vi "Wristband main - Keytap Leap based.vi"() -> ()   [LabVIEW 2014]
uses:
  Typedef/sensor_data.ctl
  Typedef/keytap_data.ctl
  Typedef/flexext_data.ctl
  SubVIs/Save Blocks - 2D.vi
  <vilib>/MakerHub/LINX/Public/Peripherals/Analog/Analog Read N Chans.vi
  <vilib>/MakerHub/LINX/LMH-LINX.lvlib
panel:
  in  "X Scale.Range:Maximum":dbl=200.0 format="%#_13g"
  in  "X Scale.Range:Minimum":dbl format="%#_13g"
  in  "X-scale change":bool
  in  "Clear Plot":bool
  in  "Acquire":bool
  in  "Tacq":u32=50 caption="Acquisition Interval" min=50 max=10000 step=50 format="%.0fms"
  in  "N pts":i32=500
  in  "Session name":string="Sessione Mat"
  in  "Save to path":path=path "C:/Users/Andrea/Desktop/Programmi LabView/Smart Wristband"
  out "Leap \nConnected?":bool caption="Leap Motion"
  in  "Arduino Port":refnum<visa-resource-name>="COM4"
  out "Status":bool=TRUE caption="Arduino"
  out "Sensor Chart":T1(graph)
  out "Grab Strength":u8
  out "Flexext cluster":T2
  out "Keytap cluster":T3={"Pollice"=5, "Indice"=5, "Medio"=5, "Anulare"=5, "Mignolo"=5}
  out "Sensor Data":T4={"Sensor  Chan 0"=1.66015625, "Sensor Chan 1"=2.060546875, "Sensor Chan 2"=2.099609375, "Sensor Chan 3"=2.12890625, "Sensor Chan 4"=2.0751953125, "Sensor Chan 5"=1.8115234375}
  in  "Exit":bool=TRUE
  out "Event Chart":T5(graph)={"Estensione"=0, "Flessione"=0, "Pollice"=5, "Indice"=5, "Medio"=5, "Anulare"=5, "Mignolo"=5, "Grab Strength"=0}
  # "Connection panel"
  # "Acquisition panel"
  # "Save settings"
  # "Connection status"
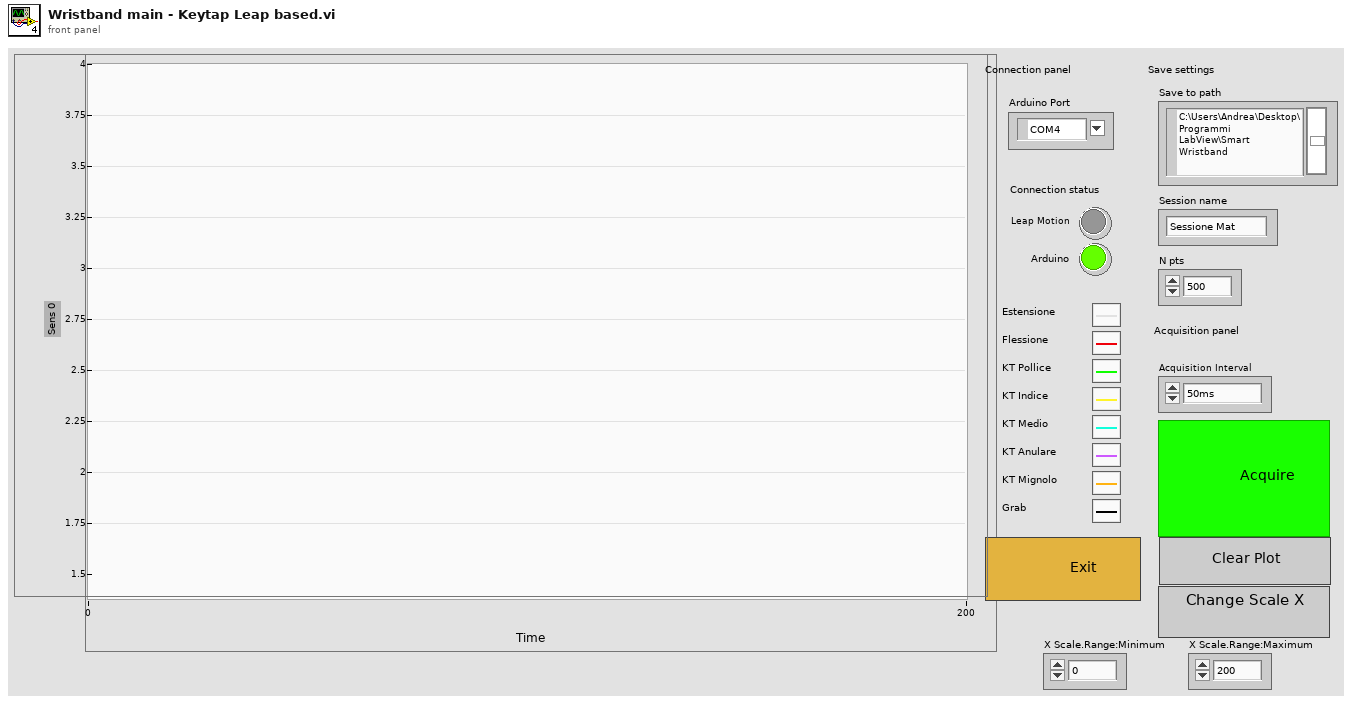
[diagram p1: front panel]
types:
  T1 = cluster{"Sensor  Chan 0":dbl, "Sensor Chan 2":dbl, "Sensor Chan 4":dbl, "Sensor Chan 5":dbl}
  T2 = typedef "flexext_data.ctl" = cluster{"Estensione":u8, "Flessione":u8}
  T3 = typedef "keytap_data.ctl" = cluster{"Pollice":u8, "Indice":u8, "Medio":u8, "Anulare":u8, "Mignolo":u8}
  T4 = typedef "Sensor_data.ctl" = cluster{"Sensor  Chan 0":dbl, "Sensor Chan 1":dbl, "Sensor Chan 2":dbl, "Sensor Chan 3":dbl, "Sensor Chan 4":dbl, "Sensor Chan 5":dbl}
  T5 = cluster{"Estensione":u8, "Flessione":u8, "Pollice":u8, "Indice":u8, "Medio":u8, "Anulare":u8, "Mignolo":u8, "Grab Strength":u8}
  T6 = typedef "LMH-LINX.lvlib/LINX Ref.ctl" = cluster{"Platform":T7, "Interface":T8, "LINX Device Config":T9}
  T7 = typedef "LMH-LINX.lvlib/Platform.ctl" = enum16{"LINX", "myRIO"}
  T8 = typedef "LMH-LINX.lvlib/Interface.ctl" = enum16{"Serial", "TCP"}
  T9 = typedef "LMH-LINX.lvlib/Device.lvlib/LINX Device Config.ctl" = cluster{"Interface":T8, "COM Port":refnum<visa-resource-name>, "TCP Configuration":T10, "Device Family":u8, "Device ID":u8, "Device Name":string, "TCP Ref":refnum<k5>, "Channels":T11}
  T10 = typedef "LMH-LINX.lvlib/Device.lvlib/TCP Config.ctl" = cluster{"IP Address":string, "Port":u16}
  T11 = typedef "LMH-LINX.lvlib/Channels.ctl" = cluster{"DI":u8[], "DO":u8[], "AI":u8[], "AO":u8[], "PWM":u8[], "QE":u8[], "UART":u8[], "I2C 2":u8[], "SPI":u8[], "CAN":u8[], "Servo":u8[], "AI Ref (V)":dbl, "AO Ref (V)":dbl, "AO Resolution (Bits)":u8}
  T12 = typedef "Leap Handle.ctl" = cluster{"LeapCSharp":refnum<k24>}
  T13 = cluster{"Estensione":u8, "Flessione":u8, "Pollice":u8, "Indice":u8, "Medio":u8, "Anulare":u8, "Mignolo":u8, "Grab Strength":u8}[]
  T14 = cluster{"Sensor  Chan 0":dbl, "Sensor Chan 2":dbl, "Sensor Chan 4":dbl, "Sensor Chan 5":dbl}[]
  T15 = cluster{"Sensor  Chan 0":dbl, "Sensor Chan 1":dbl, "Sensor Chan 2":dbl, "Sensor Chan 3":dbl}
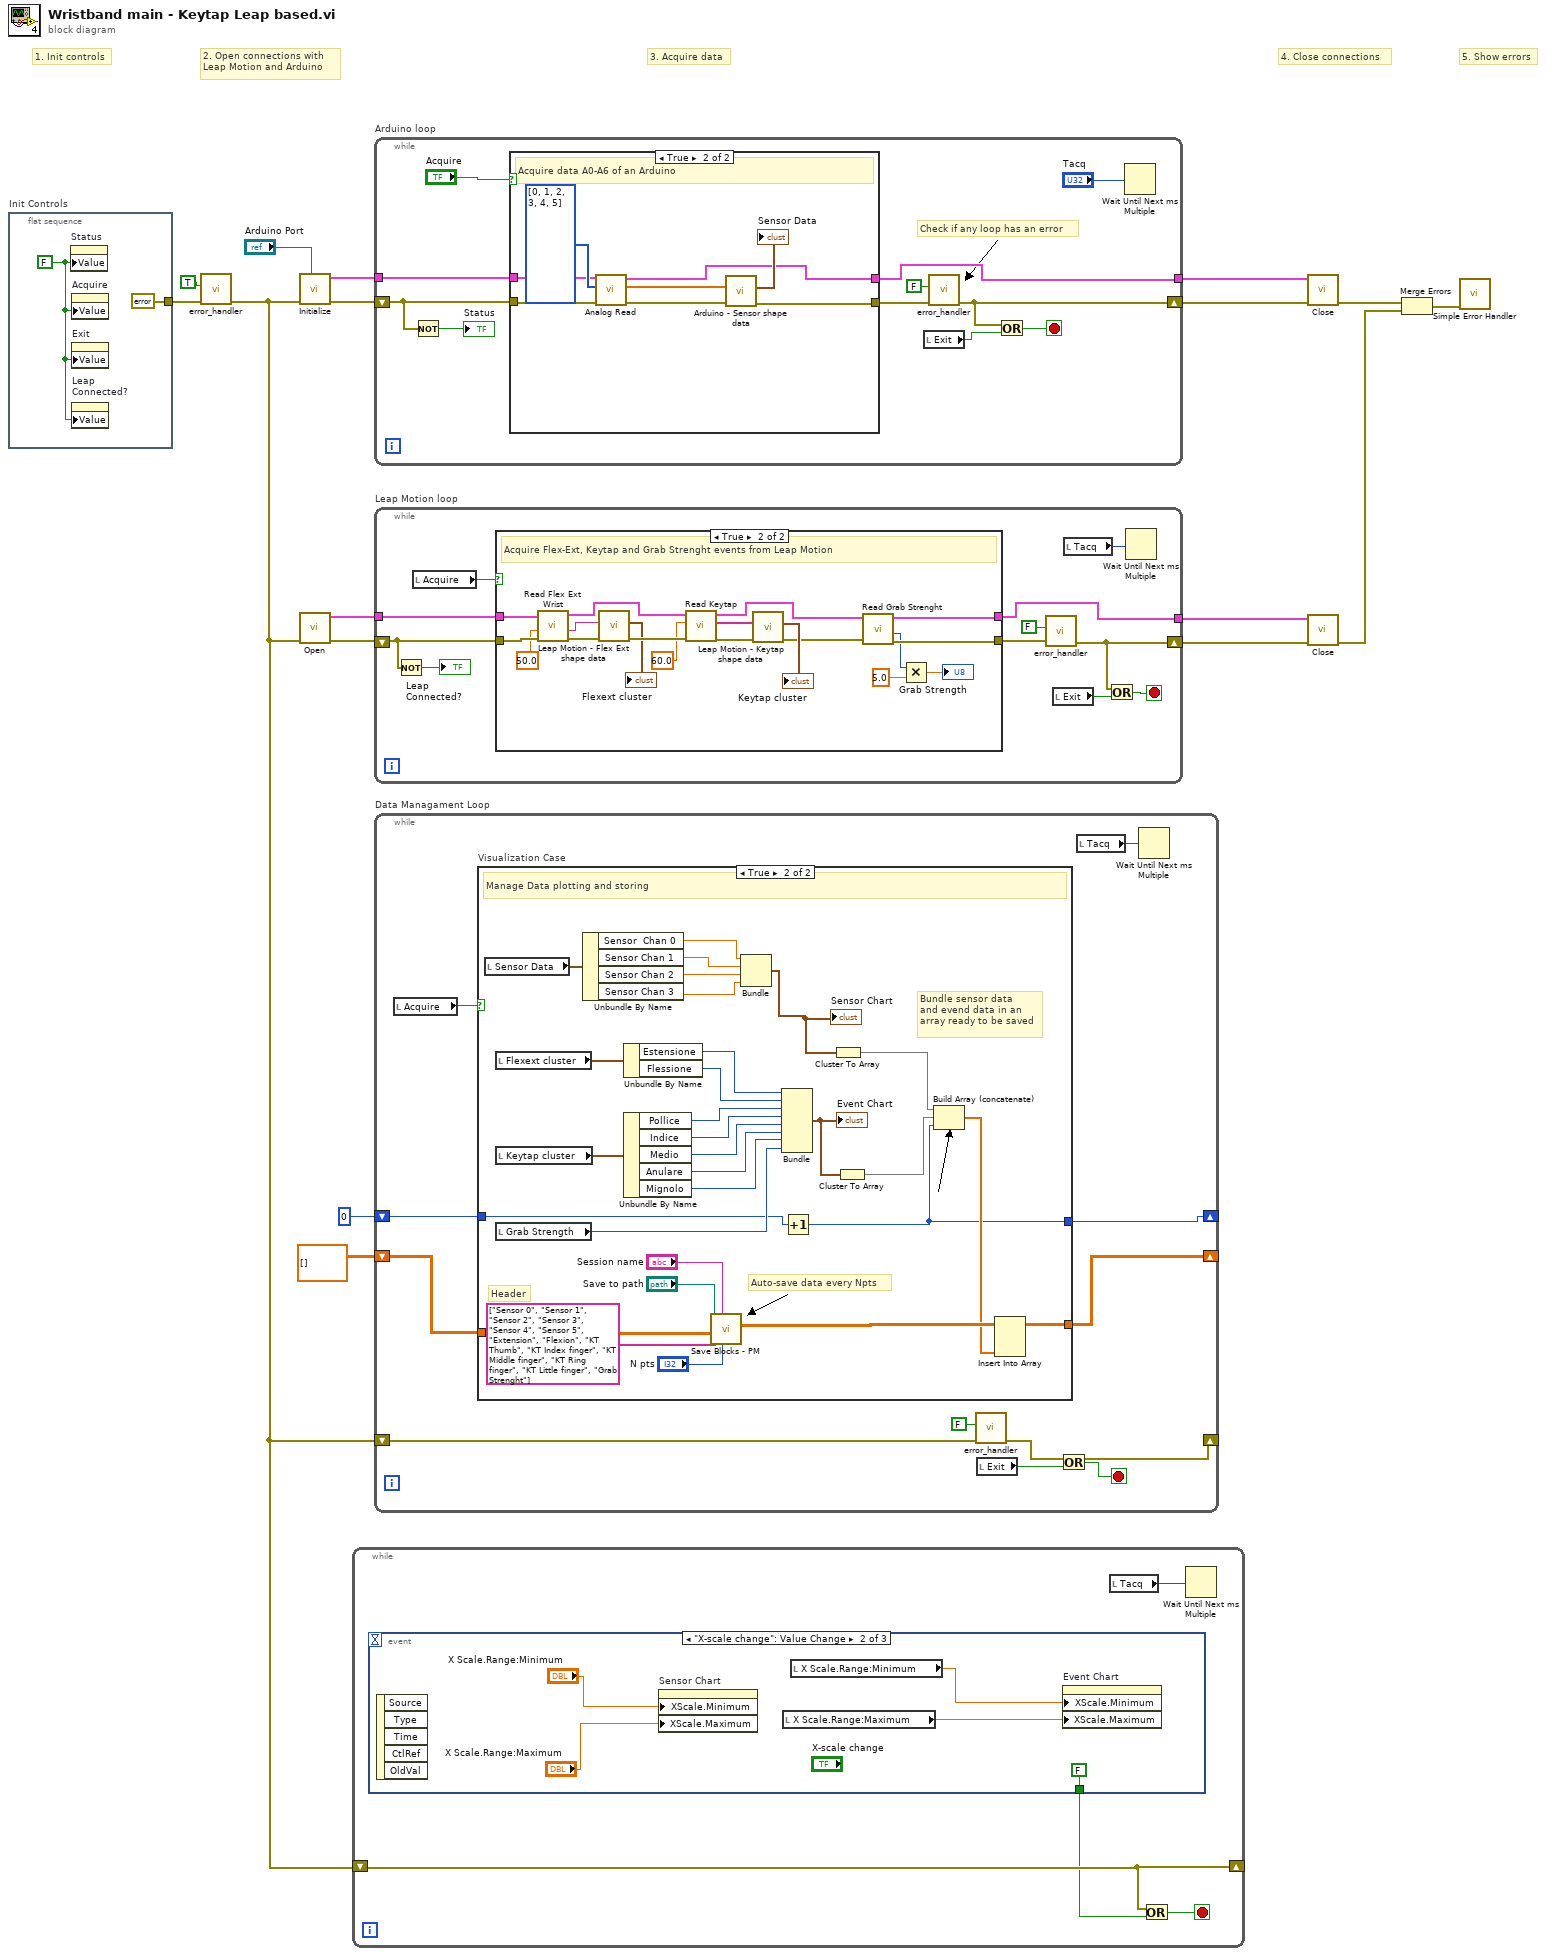
[diagram p0: block diagram]
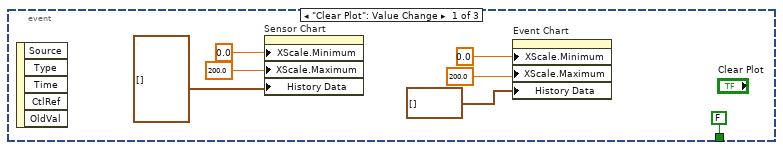
[diagram p2: hidden frame]
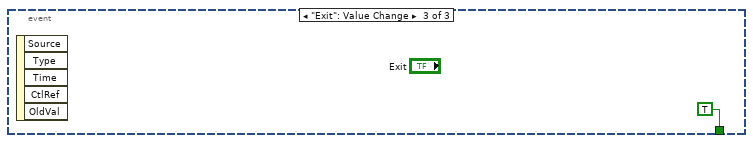
[diagram p3: hidden frame]
diagram:
  # "5. Show errors"
  # "4. Close connections"
  # "3. Acquire data"
  # "2. Open connections with\nLeap Motion and Arduino"
  # "1. Init controls"
  n1 = flat-sequence "Init Controls" {
    tunnel: [errorcluster {"status"=FALSE, "code"=0, "source"=""} ("Error In")] -> w8
    frame #0 {
      w18 = FALSE ("Status")
      n2 = property on="Status" class="Bool (strict)"("Value"=w18) -> ()  [unwired: 2 in, 2 out]
      n3 = property on="Acquire" class="Bool (strict)"("Value"=w18) -> ()  [unwired: 2 in, 2 out]
      n4 = property on="Exit" class="Bool (strict)"("Value"=w18) -> ()  [unwired: 2 in, 2 out]
      n5 = property on="Leap \nConnected?" class="Bool (strict)"("Value"=w18) -> ()  [unwired: 2 in, 2 out]
    }
  }
  n6 = call "error_handler.vi"("Error In"=w8, "Reset"=TRUE) -> ("Error Out"=w2:errorcluster)  [unwired: 9 in]
  n7 = call <vilib>:"Initialize.vi"("Serial Port"="Arduino Port", "Error In"=w2) -> ("Error Out"=w16:errorcluster, "LINX Ref"=w17:T6)  [unwired: 7 in, 1 out]
  n8 = call "Open.vi"("Error In"=w2) -> ("Error Out"=w11:errorcluster, "Leap Handle"=w12:T12)  [unwired: 9 in]
  n9 = while {
    shift-right: [w21] -> _
    shift-left: w2 -> [w21]
    stop <- w22 stop-if-true
    n10 = event shown="[1] \"X-scale change\": Value Change" {
      selector: _ -> [_ _ _]
      dyn-events: _ -> [_ _ _]
      timeout: _ -> [_ _ _]
      tunnel: [FALSE FALSE TRUE] -> w20
      event "Clear Plot": Value Change {
        n11 = event-data() -> ()  [unwired: 1 in, 5 out]
        n12 = property on="Sensor Chart" class="WFChart (strict)"("XScale.Minimum"=0.0 ("X Scale.Range:Minimum"), "XScale.Maximum"=200.0 ("X Scale.Range:Maximum"), "History Data"=T14 []) -> ()  [unwired: 2 in, 2 out]
        n13 = property on="Event Chart" class="WFChart (strict)"("XScale.Minimum"=0.0 ("X Scale.Range:Minimum"), "XScale.Maximum"=200.0 ("X Scale.Range:Maximum"), "History Data"=T13 []) -> ()  [unwired: 2 in, 2 out]
      }
      event "X-scale change": Value Change {
        n14 = event-data() -> ()  [unwired: 1 in, 5 out]
        n15 = property on="Sensor Chart" class="WFChart (strict)"("XScale.Minimum"="X Scale.Range:Minimum", "XScale.Maximum"="X Scale.Range:Maximum") -> ()  [unwired: 2 in, 2 out]
        n16 = local read "X Scale.Range:Maximum"() -> (w31:dbl)
        n17 = local read "X Scale.Range:Minimum"() -> (w34:dbl)
        n18 = property on="Event Chart" class="WFChart (strict)"("XScale.Minimum"=w34, "XScale.Maximum"=w31) -> ()  [unwired: 2 in, 2 out]
      }
      event "Exit": Value Change {
        n19 = event-data() -> ()  [unwired: 1 in, 5 out]
      }
    }
    n20 = local read "Tacq"() -> (w23:u32)
    n21 = Or(x=w21, y=w20) -> (x .or. y?=w22:bool)
    n22 = Wait Until Next ms Multiple(millisecond multiple=w23) -> ()  [unwired: 1 out]
  }
  n23 = while "Arduino loop" {
    tunnel: w17 -> [w46]
    tunnel: [w39] -> w13
    shift-right: [w40] -> w14
    shift-left: w16 -> [w43]
    stop <- w45 stop-if-true
    # "Check if any loop has an error"
    n24 = Not(x=w43) -> (.not. x?=→"Status":bool)
    n25 = case shown="True" "Acquire" {
      tunnel: w46 -> [w48 w55]
      tunnel: w43 -> [w49 w57]
      tunnel: [w48 w50] -> w39
      tunnel: [w49 w53] -> w41
      frame False {
        # "Idle"
      }
      frame True {
        # "Acquire data A0-A6 of an Arduino"
        n26 = call-poly <vilib>:"Analog Read.vi"("Error In"=w57, "AI Channel(s)"=u8[] [0, 1, 2, 3, 4, 5], "LINX Resource"=w55) -> ("Error Out"=w54:errorcluster, "Voltages"=w52:dbl[], "LINX Resource"=w50:T6)  [unwired: 5 in, 1 out]
        n27 = call "Arduino - Sensor shape data.vi"("Error In"=w54, "Sensor Data in"=w52) -> ("Error Out"=w53:errorcluster, "Sensor Data Out"=→"Sensor Data":T4)  [unwired: 8 in]
      }
    }
    n28 = local read "Exit"() -> (w37:bool)
    n29 = call "error_handler.vi"("Error In"=w41, "Reset"=FALSE) -> ("Error Out"=w40:errorcluster)  [unwired: 9 in]
    n30 = Or(x=w40, y=w37) -> (x .or. y?=w45:bool)
    n31 = Wait Until Next ms Multiple(millisecond multiple="Tacq") -> ()  [unwired: 1 out]
  }
  n32 = while "Leap Motion loop" {
    tunnel: w12 -> [w66]
    tunnel: [w60] -> w10
    shift-right: [w62] -> w9
    shift-left: w11 -> [w59]
    stop <- w67 stop-if-true
    n33 = Not(x=w59) -> (.not. x?=→"Leap \nConnected?":bool)
    n34 = local read "Acquire"() -> (w64:bool)
    n35 = case shown="True" w64 {
      tunnel: w66 -> [w70 w89]
      tunnel: w59 -> [w69 w88]
      tunnel: [w70 w76] -> w60
      tunnel: [w69 w75] -> w63
      frame False {
        # "Idle"
      }
      frame True {
        # "Acquire Flex-Ext, Keytap and Grab Strenght events from Leap Motion"
        n36 = call "Read Flex Ext Wrist.vi"("Error In"=w88, "Flex Extension threshold"=sgl 50.0, "Leap Handle In"=w89) -> ("Error Out"=w86:errorcluster, "Wrist Flextion/Extension"=w85:string, "Leap Handle Out"=w84:T12)  [unwired: 4 in]
        n37 = call "Leap Motion - Flex Ext shape data.vi"("Error In"=w86, "Event In"=w85) -> ("Error Out"=w83:errorcluster, "Flexext cluster"=→"Flexext cluster":T2)  [unwired: 8 in]
        n38 = call "Read Keytap.vi"("Error In"=w83, "Key Tap Thresh"=sgl 60.0, "Leap Handle In"=w84) -> ("Error Out"=w82:errorcluster, "Key tap"=w81:string[], "Leap Handle Out"=w78:T12)  [unwired: 3 in, 2 out]
        n39 = call "Leap Motion - Keytap shape data.vi"("Error In"=w82, "Key tap"=w81) -> ("Error Out"=w77:errorcluster, "Keytap cluster"=→"Keytap cluster":T3)  [unwired: 8 in]
        n40 = call "Read Grab Strenght.vi"("Error In"=w77, "Leap Handle In"=w78) -> ("Error Out"=w75:errorcluster, "Numeric Palm State"=w71:i32, "Leap Handle Out"=w76:T12)  [unwired: 5 in, 2 out]
        n41 = Multiply(x=w71, y=sgl 5.0) -> (x*y=→"Grab Strength":sgl)
      }
    }
    n42 = call "error_handler.vi"("Error In"=w63, "Reset"=FALSE) -> ("Error Out"=w62:errorcluster)  [unwired: 9 in]
    n43 = local read "Exit"() -> (w68:bool)
    n44 = local read "Tacq"() -> (w65:u32)
    n45 = Or(x=w62, y=w68) -> (x .or. y?=w67:bool)
    n46 = Wait Until Next ms Multiple(millisecond multiple=w65) -> ()  [unwired: 1 out]
  }
  n47 = while "Data Managament Loop" {
    shift-right: [w95] -> _
    shift-left: w2 -> [w96]
    shift-right: [w94] -> _
    shift-left: dbl[][] [] -> [w93]
    shift-right: [w90] -> _
    shift-left: 0 -> [w91]
    stop <- w97 stop-if-true
    n48 = local read "Acquire"() -> (w100:bool)
    n49 = case "Visualization Case" shown="True" w100 {
      tunnel: [w102 w114] -> w94
      tunnel: w93 -> [w102 w112]
      tunnel: w91 -> [w101 w104]
      tunnel: [w101 w103] -> w90
      frame False {
        # "Idle"
      }
      frame True {
        # "Header"
        # "Auto-save data every Npts"
        # "Bundle sensor data\nand evend data in an\narray ready to be saved"
        # "Manage Data plotting and storing"
        n50 = local read "Sensor Data"() -> (w110:T4)
        n51 = local read "Flexext cluster"() -> (w131:T2)
        n52 = local read "Keytap cluster"() -> (w130:T3)
        n53 = local read "Grab Strength"() -> (w122:u8)
        n54 = Unbundle By Name(w110) -> ("Sensor  Chan 0"=w109:dbl, "Sensor Chan 1"=w108:dbl, "Sensor Chan 2"=w107:dbl, "Sensor Chan 3"=w106:dbl)
        n55 = Unbundle By Name(w131) -> ("Estensione"=w129:u8, "Flessione"=w128:u8)
        n56 = Unbundle By Name(w130) -> ("Pollice"=w127:u8, "Indice"=w126:u8, "Medio"=w125:u8, "Anulare"=w124:u8, "Mignolo"=w123:u8)
        n57 = call-poly "Save Blocks - PM.vi"("N pts"="N pts", "Session name"="Session name", "2D Data In"=w112, "Column headers"=string[] ["Sensor 0", "Sensor 1", "Sensor 2", "Sensor 3", "Sensor 4", "Sensor 5", "Extension", "Flexion", "KT Thumb", "KT Index finger", "KT Middle finger", "KT Ring finger", "KT Little finger", "Grab Strenght"], "Save to path"="Save to path") -> ("2D Data Out"=w118:dbl[][])  [unwired: 5 in, 1 out]
        n58 = Bundle("Sensor  Chan 0"=w109, "Sensor Chan 1"=w108, "Sensor Chan 2"=w107, "Sensor Chan 3"=w106) -> (w105:T15)  [unwired: 1 in]
        "Sensor Chart" <- w105
        n59 = Bundle("Estensione"=w129, "Flessione"=w128, "Pollice"=w127, "Indice"=w126, "Medio"=w125, "Anulare"=w124, "Mignolo"=w123, "Grab Strength"=w122) -> (w121:T5)  [unwired: 1 in]
        "Event Chart" <- w121
        n60 = Increment(x=w104) -> (x+1=w103:i32)
        n61 = Cluster To Array(cluster=w105) -> (array=w120:dbl[])
        n62 = Cluster To Array(cluster=w121) -> (array=w119:u8[])
        n63 = Build Array (concatenate)(w120, w119, w103) -> (w113:dbl[])
        n64 = Insert Into Array(array=w118, new element=w113) -> (w114:dbl[][])  [unwired: 2 in]
      }
    }
    n65 = call "error_handler.vi"("Error In"=w96, "Reset"=FALSE) -> ("Error Out"=w95:errorcluster)  [unwired: 9 in]
    n66 = local read "Exit"() -> (w98:bool)
    n67 = Or(x=w95, y=w98) -> (x .or. y?=w97:bool)
    n68 = local read "Tacq"() -> (w92:u32)
    n69 = Wait Until Next ms Multiple(millisecond multiple=w92) -> ()  [unwired: 1 out]
  }
  n70 = call <vilib>:"Close.vi"("Error In"=w14, "LINX Resource"=w13) -> ("Error Out"=w5:errorcluster)  [unwired: 8 in, 1 out]
  n71 = call <vilib>:"Close.vi"("Error In"=w9, "Leap Handle"=w10) -> ("Error Out"=w4:errorcluster)  [unwired: 9 in]
  n72 = Merge Errors(w5, w4) -> (w6:errorcluster)
  n73 = call <vilib>:"Simple Error Handler.vi"("error in (no error)"=w6) -> ()  [unwired: 4 in, 5 out]
